vi "Write Publish Topic.vi"(8 "error in (no error)":errorcluster, 10 "Publish Topic":string, 11 "SystemLinkOutputTerminal in":refnum<class "SystemLinkOutputTerminal.lvclass">) -> (0 "error out":errorcluster, 3 "SystemLinkOutputTerminal out":refnum<class "SystemLinkOutputTerminal.lvclass">)   [LabVIEW 2016, in "SystemLinkOutputTerminal.lvclass"]
uses:
  SystemLinkOutputTerminal.lvclass
  SystemLinkOutputTerminal.lvclass/SystemLinkOutputTerminal.ctl
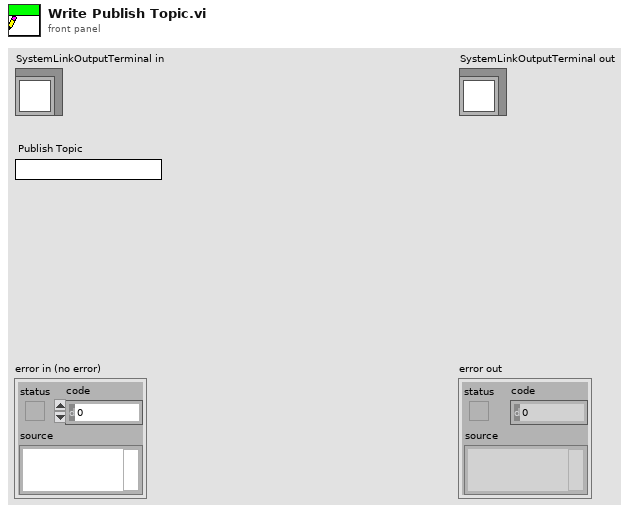
[diagram p1: front panel]
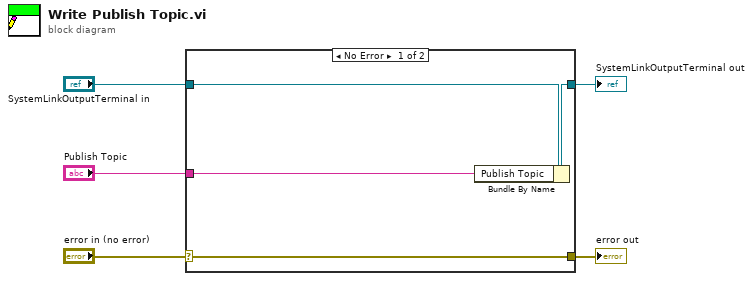
[diagram p0: block diagram]
diagram:
  n1 = case shown="No Error" "error in (no error)" {
    selector: "error in (no error)" -> [w9 w10]
    tunnel: [w9 w10] -> w4
    tunnel: [w7 w11] -> w2
    tunnel: "SystemLinkOutputTerminal in" -> [w8 w11]
    tunnel: "Publish Topic" -> [w6 _]
    frame No Error {
      n2 = Bundle By Name(cluster=w8, "Publish Topic"=w6) -> (w7:refnum<class "SystemLinkOutputTerminal.lvclass">)
    }
    frame Error {
    }
  }
  "error out" <- w4
  "SystemLinkOutputTerminal out" <- w2
